vi "tcp.vi"() -> ()   [LabVIEW 2020]
uses:
  <vilib>/regexp/Match Regular Expression.xnode
panel:
  out "data out 2":string
  out "code 2":i32
  out "Waveform Chart":dbl(graph)
  in  "stop 4":bool
  out "Ostatnia 2":string
  out "data out":string
  out "code":i32
  in  "stop 3":bool
  out "Ostatnia":string
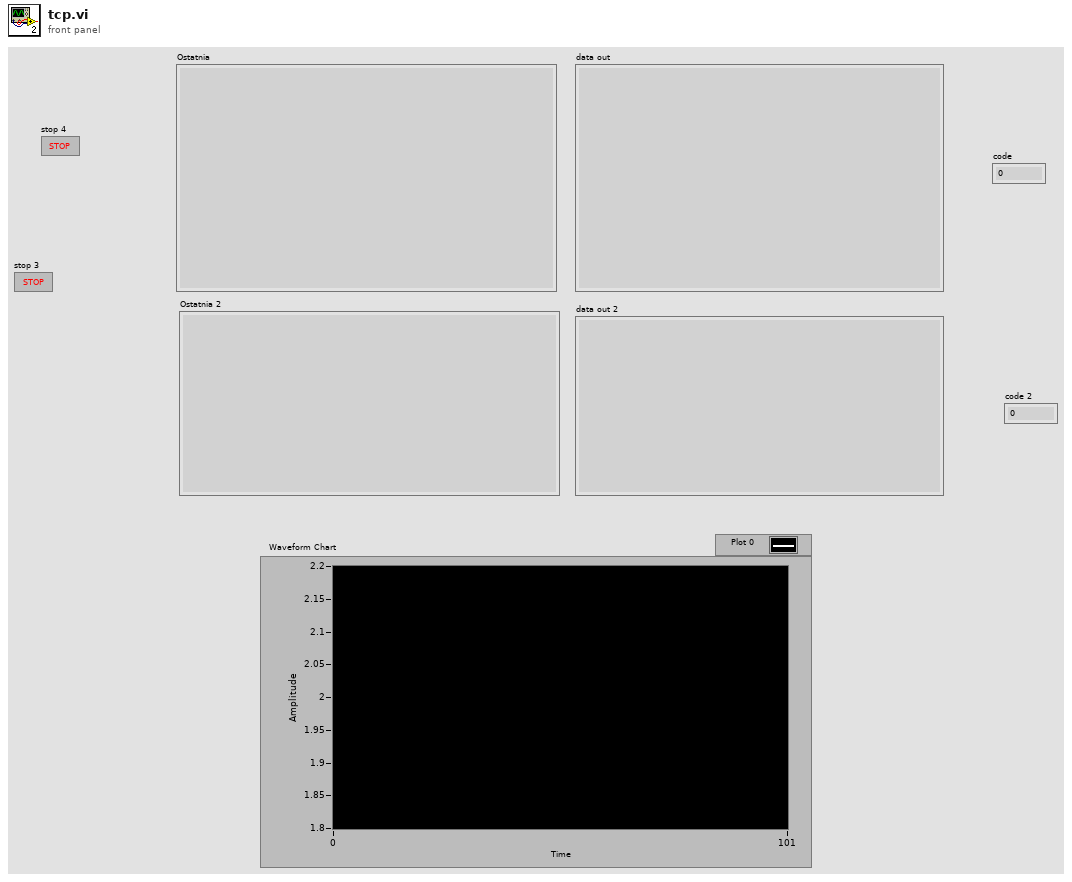
[diagram p1: front panel]
types:
  T1 = enum16{"Standard", "Buffered", "CRLF", "Immediate"}
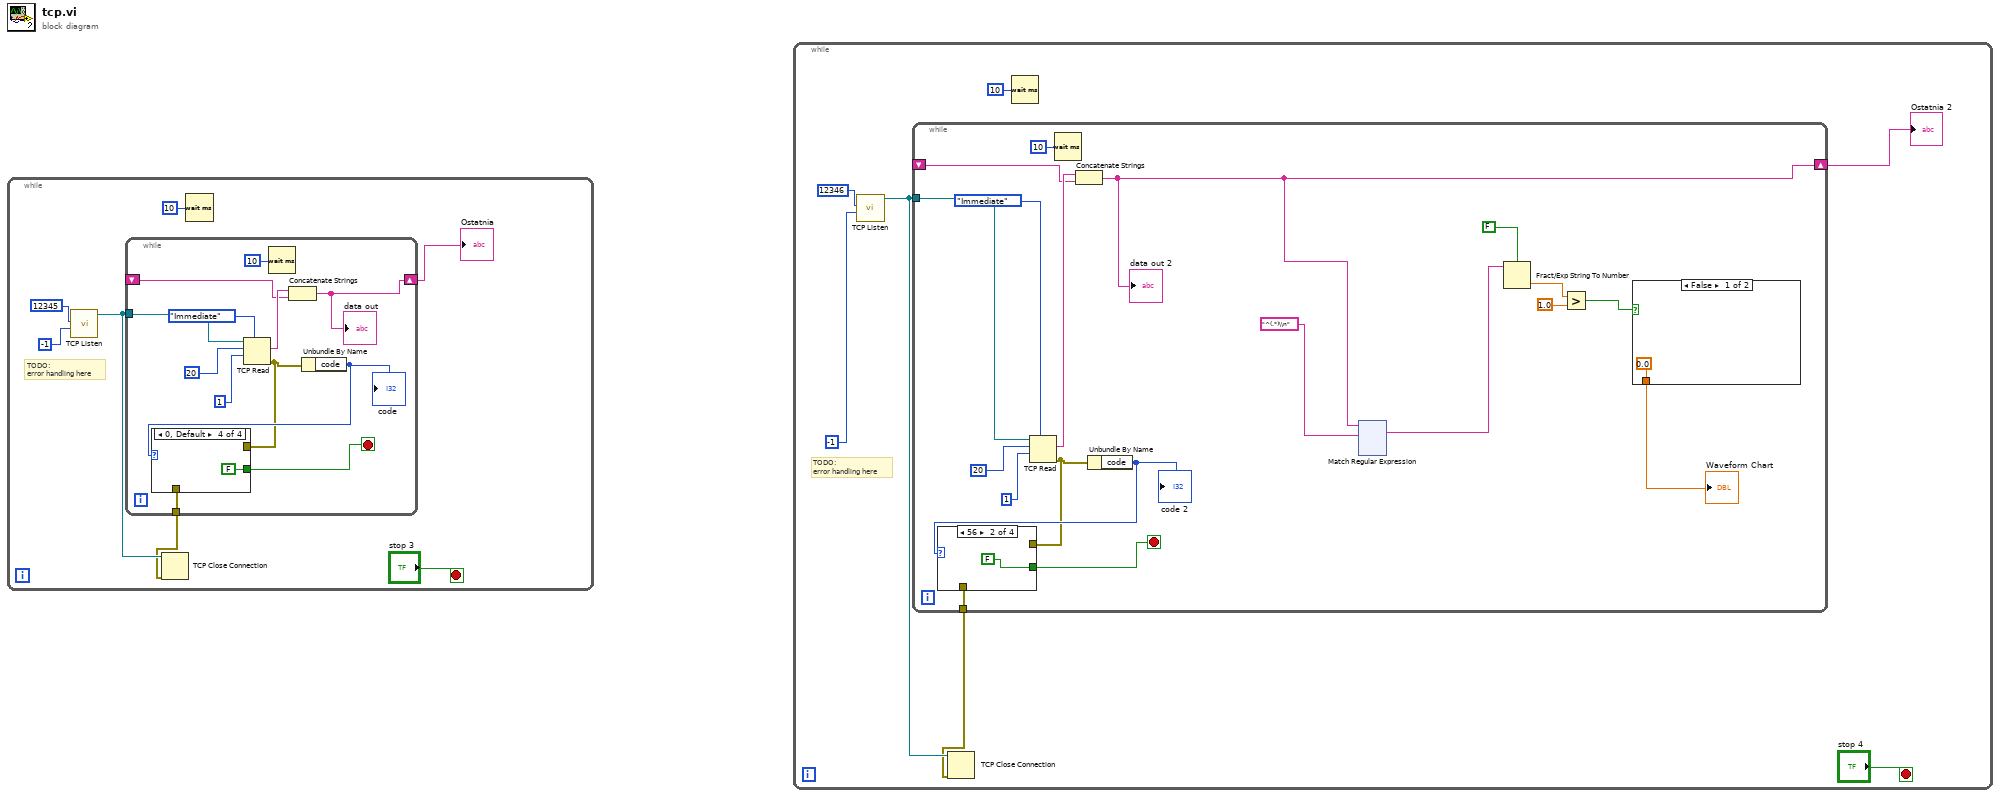
[diagram p0: block diagram]
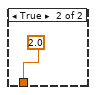
[diagram p2: hidden frame]
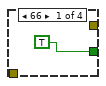
[diagram p3: hidden frame]
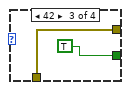
[diagram p4: hidden frame]
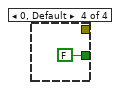
[diagram p5: hidden frame]
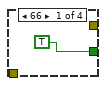
[diagram p6: hidden frame]
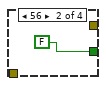
[diagram p7: hidden frame]
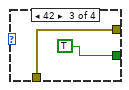
[diagram p8: hidden frame]
diagram:
  n1 = while {
    stop <- "stop 3" stop-if-true
    # "TODO:\nerror handling here"
    n2 = call <vilib>:"TCP Listen.vi"("timeout ms (wait forever: -1)"=-1, "port"=u16 12345) -> ("connection ID"=w7:refnum<k5>)  [unwired: 5 in, 4 out]
    n3 = while {
      tunnel: w7 -> [w17]
      shift-right: [w14] -> w2
      shift-left: _ -> [w15]
      tunnel: [w10] -> w4
      stop <- w12 stop-if-true
      n4 = TCP Read(connection ID=w17, bytes to read=20, 7:T1."Immediate" ("mode (standard)"), 9:1 ("timeout ms (25000)")) -> (data out=w16:string, error out=w11:errorcluster)  [unwired: 1 in, 1 out]
      n5 = Wait (ms)(milliseconds to wait=u32 10) -> ()  [unwired: 1 out]
      n6 = Concatenate Strings(w16, w15) -> (w14:string)
      "data out" <- w14
      n7 = Unbundle By Name(w11) -> ("code"=w13:i32)
      "code" <- w13
      n8 = case shown="0, Default" w13 {
        tunnel: [TRUE FALSE TRUE FALSE] -> w12
        tunnel: w11 -> [_ _ w22 _]
        tunnel: [_ _ w22 _] -> w10
        frame 66 {
        }
        frame 56 {
        }
        frame 42 {
        }
        frame 0, Default {
        }
      }
    }
    "Ostatnia" <- w2
    n9 = TCP Close Connection(connection ID=w7, error in (no error)=w4) -> ()  [unwired: 1 in, 2 out]
    n10 = Wait (ms)(milliseconds to wait=u32 10) -> ()  [unwired: 1 out]
  }
  n11 = while {
    stop <- "stop 4" stop-if-true
    # "TODO:\nerror handling here"
    n12 = call <vilib>:"TCP Listen.vi"("timeout ms (wait forever: -1)"=-1, "port"=u16 12346) -> ("connection ID"=w31:refnum<k5>)  [unwired: 5 in, 4 out]
    n13 = while {
      tunnel: w31 -> [w48]
      shift-right: [w36] -> w25
      shift-left: _ -> [w46]
      tunnel: [w42] -> w28
      stop <- w44 stop-if-true
      n14 = TCP Read(connection ID=w48, bytes to read=20, 7:T1."Immediate" ("mode (standard)"), 9:1 ("timeout ms (25000)")) -> (data out=w47:string, error out=w43:errorcluster)  [unwired: 1 in, 1 out]
      n15 = Wait (ms)(milliseconds to wait=u32 10) -> ()  [unwired: 1 out]
      n16 = Concatenate Strings(w47, w46) -> (w36:string)
      "data out 2" <- w36
      n17 = Unbundle By Name(w43) -> ("code"=w45:i32)
      "code 2" <- w45
      n18 = case shown="56" w45 {
        tunnel: [TRUE FALSE TRUE FALSE] -> w44
        tunnel: w43 -> [_ _ w172 _]
        tunnel: [_ _ w172 _] -> w42
        frame 66 {
        }
        frame 56 {
        }
        frame 42 {
        }
        frame 0, Default {
        }
      }
      n19 = xnode "Match Regular Expression"("input string"=w36, "regular expression"="^(.*)\\n") -> ("whole match"=w39:string)  [unwired: 4 in, 4 out]
      n20 = Fract/Exp String To Number(use system decimal point (T)=FALSE, string=w39) -> (number=w33:dbl)  [unwired: 2 in, 1 out]
      n21 = Greater?(x=w33, y=1.0) -> (0:w35:bool)
      n22 = case shown="False" w35 {
        tunnel: [0.0 2.0] -> w32
        frame False {
        }
        frame True {
        }
      }
      "Waveform Chart" <- w32
    }
    "Ostatnia 2" <- w25
    n23 = TCP Close Connection(connection ID=w31, error in (no error)=w28) -> ()  [unwired: 1 in, 2 out]
    n24 = Wait (ms)(milliseconds to wait=u32 10) -> ()  [unwired: 1 out]
  }
